vi "Rename Illegal Characters to Wavename.vi"(1 "Wavename":string) -> (0 "Command string":string)   [LabVIEW 2016, in "LVtoITX.lvclass"]
uses:
  LVtoITX.lvclass
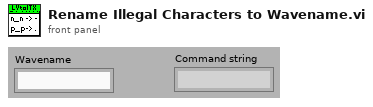
[diagram p1: front panel]
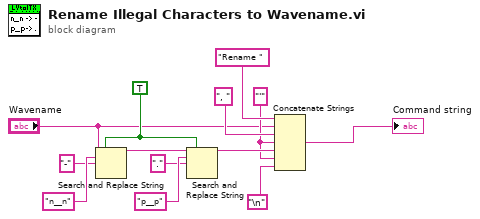
[diagram p0: block diagram]
diagram:
  w3 = "'" ("search string")
  w5 = TRUE ("replace all? (F)")
  n1 = Search and Replace String(replace all?=w5, input string="Wavename", search string="n__n" ("replace string (\"\")"), replace string="-" ("search string")) -> (result string=w12:string)  [unwired: 4 in, 3 out]
  n2 = Search and Replace String(replace all?=w5, input string=w12, search string="p__p" ("replace string (\"\")"), replace string="." ("search string")) -> (result string=w4:string)  [unwired: 4 in, 3 out]
  n3 = Concatenate Strings("Rename " ("string"), "Wavename", ", " ("search string"), w3, w4, w3, "\n") -> (→"Command string":string)
